vi "15-10-5-2.vi"() -> ()   [LabVIEW 2025]
uses:
  <vilib>/Platform/TimedLoop/XDataNode/timing_clust.ctl
  <vilib>/Platform/TimedLoop/XDataNode/nitl_modes.ctl
  <vilib>/Platform/TimedLoop/XDataNode/wakeup.ctl
  <vilib>/rvi/Emulation/niFpgaSctlEmulationGetInTimedLoop.vi
  <vilib>/rvi/Emulation/niFpgaEmulationReportErrorSimple.vi
  <vilib>/rvi/Emulation/niFpgaGetClockAttributes.vi
  <vilib>/rvi/Emulation/niFpgaCriticalErrorInLSC.vi
  <vilib>/rvi/linearAlgebra/MatrixMultiply/simVIs/SubVI/nifxpla_MatrixMultiply_SimMatrixSizes.vi
  <vilib>/rvi/linearAlgebra/MatrixMultiply/simVIs/SubVI/nifxpla_MatrixMultiply_Sim4WireAdapterVector.vi
  <vilib>/rvi/linearAlgebra/MatrixMultiply/simVIs/SubVI/nifxpla_MatrixMultiply_SimFrameHandShake.vi
  <vilib>/rvi/linearAlgebra/MatrixMultiply/simVIs/SubVI/nifxpla_MatrixMultiply_SimEndlessCounter.vi
  <vilib>/rvi/linearAlgebra/MatrixMultiply/simVIs/SubVI/nifxpla_MatrixMultiply_SimVectorDataBuffer.vi
  <vilib>/rvi/ClientSDK/Core/DevComputerLib/Private/Multiply(dfxp64).vi
  <vilib>/rvi/ClientSDK/Core/DevComputerLib/Private/Dfxp128ToDfxp256.vi
  <vilib>/rvi/ClientSDK/Core/DevComputerLib/Private/Add(dfxp256).vi
  <vilib>/rvi/ClientSDK/Core/DevComputerLib/Private/Subtract(dfxp256).vi
  <vilib>/rvi/ClientSDK/Core/DevComputerLib/Private/ToDfxp64(dfxp256).vi
  <vilib>/platform/TimedLoop/XDataNode/XDataNode.xnode
  <vilib>/rvi/linearAlgebra/MatrixMultiply/XNode/nifxpla_MatrixMultiply.xnode
  <vilib>/rvi/linearAlgebra/MatrixMultiply/simVIs/nifxpla_MatrixMultiply_SimTemplateEinEout.vi
  <vilib>/rvi/linearAlgebra/MatrixMultiply/simVIs/nifxpla_MatrixMultiply_SimTemplateEinVout.vi
  <vilib>/rvi/linearAlgebra/MatrixMultiply/simVIs/nifxpla_MatrixMultiply_SimTemplateVinEout.vi
  <vilib>/rvi/linearAlgebra/MatrixMultiply/simVIs/nifxpla_MatrixMultiply_SimTemplateVinVout.vi
  <vilib>/Platform/TimedLoop/XDataNode/XDNodeRunTimeDep.lvlib
panel:
  out "Latency":u32
  out "Cycle Count 3":i32
  out "C3":fxp<+/-,32,16>[](array[numeric])
  out "C3+B":fxp<+/-,33,17>[](array[numeric])
  out "Cycle Count 2":i32
  out "C2":fxp<+/-,32,16>[](array[numeric])
  out "C2+B":fxp<+/-,33,17>[](array[numeric])
  out "Cycle Count":i32
  out "C1":fxp<+/-,32,16>[](array[numeric])
  out "C1+B":fxp<+/-,33,17>[](array[numeric])
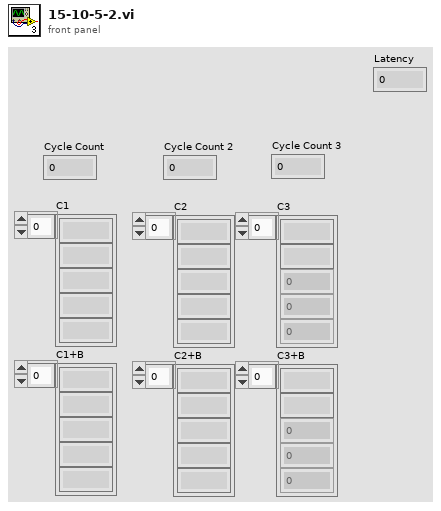
[diagram p1: front panel]
types:
  T1 = typedef "XDNodeRunTimeDep.lvlib/timing_clust.ctl" = cluster{"Expected End [f-1]":u64, "Actual End [f-1]":u64, "Finished Late? [f-1]":bool, "Expected End [i-1]":u64, "Actual End [i-1]":u64, "Finished Late? [i-1]":bool, "Expected Start [i]":u64, "Actual Start [i]":u64, "Expected Start [f]":u64, "Actual Start [f]":u64, "Source Name":string, "Structure Name":string, "Period":i64, "Deadline":i64, "Offset":i64, "Start":i64, "Priority":i32, "Timeout":i32, "Mode":T2, "Wakeup Reason":T3, "Error":errorcluster, "Source Type":string, "Secondary Source Type":string, "Global End Time":u64, "Global Start Time":u64, "Frame Duration":u64, "Iteration Duration":u64, "Assigned CPU":i32, "I/O Scan Engine Mode":u32}
  T2 = typedef "XDNodeRunTimeDep.lvlib/nitl_modes.ctl" = enum32{"No Change", "Process missed periods, maintain original phase", "Discard missed periods, maintain original phase", "Process missed periods, ignore original phase", "Discard missed periods, ignore original phase"}
  T3 = typedef "XDNodeRunTimeDep.lvlib/wakeup.ctl" = enum32{"Normal", "Aborted", "Asynchronous wakeup", "Timing source error", "Timed loop error", "Timeout"}
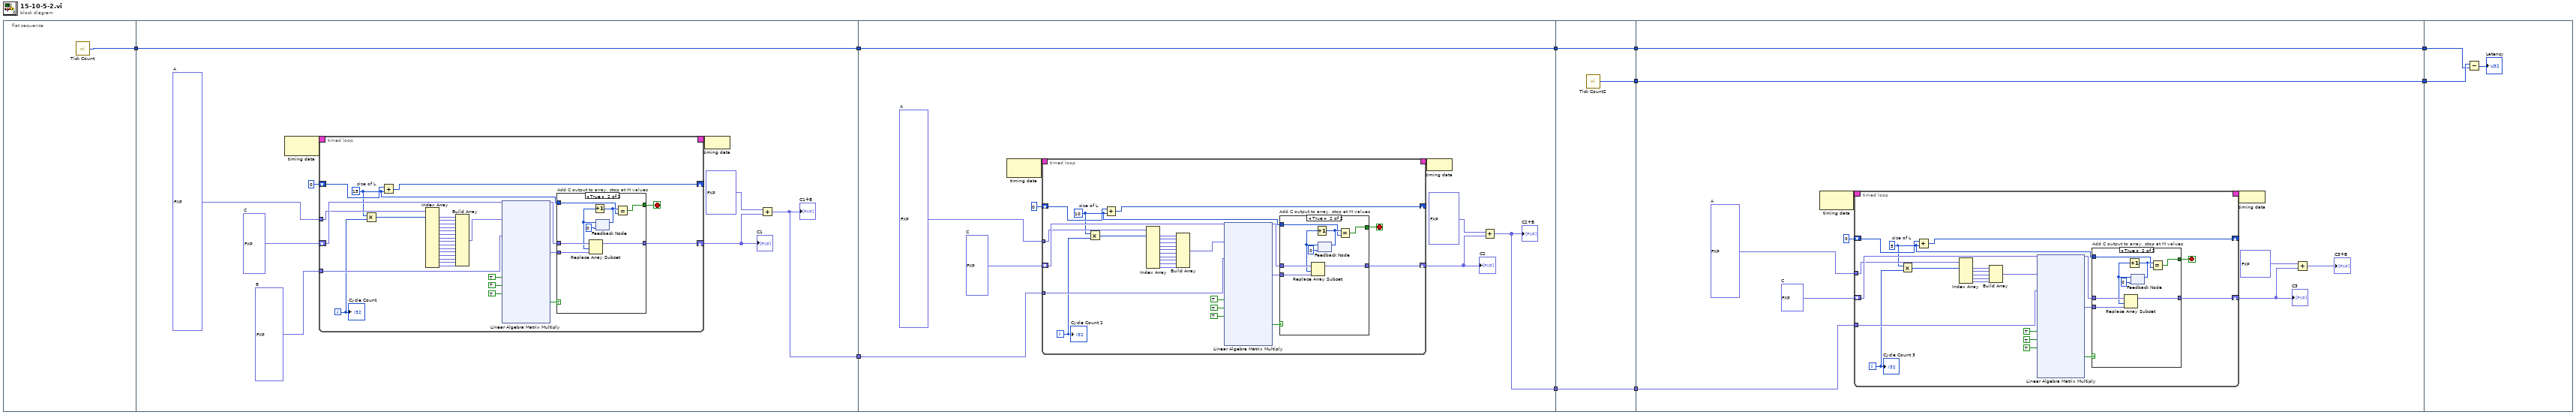
[diagram p0: block diagram]
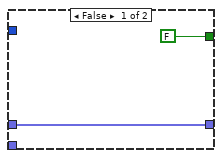
[diagram p2: hidden frame]
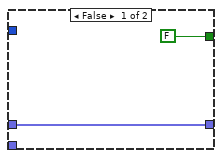
[diagram p3: hidden frame]
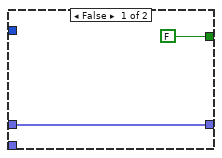
[diagram p4: hidden frame]
diagram:
  n1 = flat-sequence {
    tunnel: [w11] -> w10
    tunnel: [w13] -> w9
    tunnel: [w12] -> w8
    tunnel: w10 -> [w12]
    tunnel: w9 -> [w69]
    tunnel: [w68] -> w7
    tunnel: w8 -> [w67]
    tunnel: [w67] -> w6
    tunnel: w7 -> [w119]
    tunnel: [w119] -> w5
    tunnel: w6 -> [w118]
    tunnel: [w118] -> w4
    tunnel: [w117] -> w3
    tunnel: w5 -> [w122]
    tunnel: w4 -> [w121]
    tunnel: [w121] -> w2
    tunnel: [w120] -> w1
    tunnel: w3 -> [w120]
    tunnel: w2 -> [w167]
    tunnel: w1 -> [w168]
    frame #0 {
      n2 = call "Tick Count"() -> ("Tick Count(Ticks)"=w11:u32)
    }
    frame #1 {
      w17 = fxp<+/-,32,16>[] [0.0, 0.0, 0.0, 0.0, 0.0, 0.0, 0.0, 0.0, 0.0, 0.0, 0.0, 0.0, 0.0, 0.0, 0.0, 0.0, 0.0, 0.0, 0.0, 0.0, 0.0, 0.0, 0.0, 0.0, 0.0, 0.0, 0.0, 0.0, 0.0, 0.0, 0.0, 0.0, 0.0, 0.0, 0.0, 0.0, 0.0, 0.0, 0.0, 0.0, 0.0, 0.0, 0.0, 0.0, 0.0, 0.0, 0.0, 0.0, 0.0, 0.0, 0.0, 0.0, 0.0, 0.0, 0.0, 0.0, 0.0, 0.0, 0.0, 0.0, 0.0, 0.0, 0.0, 0.0, 0.0, 0.0, 0.0, 0.0, 0.0, 0.0, 0.0, 0.0, 0.0, 0.0, 0.0, 0.0, 0.0, 0.0, 0.0, 0.0, 0.0, 0.0, 0.0, 0.0, 0.0, 0.0, 0.0, 0.0, 0.0, 0.0, 0.0, 0.0, 0.0, 0.0, 0.0, 0.0, 0.0, 0.0, 0.0, 0.0, 0.0, 0.0, 0.0, 0.0, 0.0, 0.0, 0.0, 0.0, 0.0, 0.0, 0.0, 0.0, 0.0, 0.0, 0.0, 0.0, 0.0, 0.0, 0.0, 0.0, 0.0, 0.0, 0.0, 0.0, 0.0, 0.0, 0.0, 0.0, 0.0, 0.0, 0.0, 0.0, 0.0, 0.0, 0.0, 0.0, 0.0, 0.0, 0.0, 0.0, 0.0, 0.0, 0.0, 0.0, 0.0, 0.0, 0.0, 0.0, 0.0, 0.0]  # A
      w18 = fxp<+/-,32,16>[] [0.0, 0.0, 0.0, 0.0, 0.0, 0.0, 0.0, 0.0, 0.0, 0.0, 0.0, 0.0, 0.0, 0.0, 0.0]  # B
      w19 = fxp<+/-,32,16>[] [0.0, 0.0, 0.0, 0.0, 0.0, 0.0, 0.0, 0.0, 0.0, 0.0]  # C
      n3 = node-c288() -> (w21:T1)  [unwired: 1 in]
      n4 = timed-loop {
        timing: w21 -> [_]
        timing-out: [_] -> w20
        shift-right: [w51] -> w15
        shift-left: w19 -> [w50]
        tunnel: w18 -> [w47]
        tunnel: w17 -> [w30]
        shift-right: [w43] -> _
        shift-left: 0 ("length") -> [w44]
        i -> [w29]
        stop <- w49 stop-if-true
        w28 = 15  # size of L
        n5 = Multiply(x=w28, y=w29) -> (x*y=w41:i32)
        n6 = Add(x=w44, y=w28) -> (x+y=w43:i32)
        n7 = Index Array(array=w30, index #1=w41) -> (element #1=w40:fxp<+/-,32,16>, element #2=w39:fxp<+/-,32,16>, element #3=w38:fxp<+/-,32,16>, element #4=w37:fxp<+/-,32,16>, element #5=w36:fxp<+/-,32,16>, element #6=w35:fxp<+/-,32,16>, element #7=w34:fxp<+/-,32,16>, element #8=w33:fxp<+/-,32,16>, element #9=w32:fxp<+/-,32,16>, element #10=w31:fxp<+/-,32,16>, element #11=w26:fxp<+/-,32,16>, element #12=w25:fxp<+/-,32,16>, element #13=w24:fxp<+/-,32,16>, element #14=w23:fxp<+/-,32,16>, element #15=w22:fxp<+/-,32,16>)  [unwired: 14 in]
        n8 = Build Array(w40, w39, w38, w37, w36, w35, w34, w33, w32, w31, w26, w25, w24, w23, w22) -> (w27:fxp<+/-,32,16>[])
        n9 = xnode ("Linear Algebra Matrix Multiply")("ar"=w27, "br"=w47, "a valid"=TRUE, "b valid"=TRUE, "ready for output (T)"=TRUE) -> ("cr"=w46:fxp<+/-,64,36>[], "output valid"=w42:bool)  [unwired: 2 in, 4 out]
        n10 = case "Add C output to array, stop at M values" shown="True" w42 {
          tunnel: w46 -> [_ w58]
          tunnel: [w54 w61] -> w51
          tunnel: w50 -> [w54 w62]
          tunnel: [FALSE w59] -> w49
          tunnel: w28 -> [_ w55]
          frame False {
          }
          frame True {
            n11 = feedback #1(0 ("x")) -> (w57:i32)
            n12 = Replace Array Subset(array=w62, new element=w58, index=w57) -> (w61:fxp<+/-,32,16>[])
            n13 = Increment(x=w57) -> (x+1=w56:i32)
            n14 = feedback-in #1(w56) -> ()
            n15 = Equal?(x=w56, y=w55) -> (x = y?=w59:bool)
          }
        }
        "Cycle Count" <- w29
      }
      "C1" <- w15
      n16 = node-c288(w20) -> ()
      n17 = Add(x=fxp<+/-,32,16>[] [0.5, 0.5, 0.5, 0.5, 0.5, 0.0, 0.0, 0.0, 0.0, 0.0], y=w15) -> (x+y=w13:fxp<+/-,33,17>[])
      "C1+B" <- w13
    }
    frame #2 {
      w73 = fxp<+/-,32,16>[] [0.0, 0.0, 0.0, 0.0, 0.0, 0.0, 0.0, 0.0, 0.0, 0.0, 0.0, 0.0, 0.0, 0.0, 0.0, 0.0, 0.0, 0.0, 0.0, 0.0, 0.0, 0.0, 0.0, 0.0, 0.0, 0.0, 0.0, 0.0, 0.0, 0.0, 0.0, 0.0, 0.0, 0.0, 0.0, 0.0, 0.0, 0.0, 0.0, 0.0, 0.0, 0.0, 0.0, 0.0, 0.0, 0.0, 0.0, 0.0, 0.0, 0.0]  # A
      w74 = fxp<+/-,32,16>[] [0.0, 0.0, 0.0, 0.0, 0.0]  # C
      n18 = node-c288() -> (w76:T1)  [unwired: 1 in]
      n19 = timed-loop {
        timing: w76 -> [_]
        timing-out: [_] -> w75
        shift-right: [w101] -> w71
        shift-left: w74 -> [w100]
        tunnel: w69 -> [w97]
        tunnel: w73 -> [w85]
        shift-right: [w93] -> _
        shift-left: 0 ("length") -> [w94]
        i -> [w84]
        stop <- w99 stop-if-true
        w83 = 10  # size of L
        n20 = Multiply(x=w83, y=w84) -> (x*y=w91:i32)
        n21 = Add(x=w94, y=w83) -> (x+y=w93:i32)
        n22 = Index Array(array=w85, index #1=w91) -> (element #1=w90:fxp<+/-,32,16>, element #2=w89:fxp<+/-,32,16>, element #3=w88:fxp<+/-,32,16>, element #4=w87:fxp<+/-,32,16>, element #5=w86:fxp<+/-,32,16>, element #6=w81:fxp<+/-,32,16>, element #7=w80:fxp<+/-,32,16>, element #8=w79:fxp<+/-,32,16>, element #9=w78:fxp<+/-,32,16>, element #10=w77:fxp<+/-,32,16>)  [unwired: 9 in]
        n23 = Build Array(w90, w89, w88, w87, w86, w81, w80, w79, w78, w77) -> (w82:fxp<+/-,32,16>[])
        n24 = xnode ("Linear Algebra Matrix Multiply")("ar"=w82, "br"=w97, "a valid"=TRUE, "b valid"=TRUE, "ready for output (T)"=TRUE) -> ("cr"=w96:fxp<+/-,64,37>[], "output valid"=w92:bool)  [unwired: 2 in, 4 out]
        n25 = case "Add C output to array, stop at M values" shown="True" w92 {
          tunnel: w96 -> [_ w108]
          tunnel: [w104 w111] -> w101
          tunnel: w100 -> [w104 w112]
          tunnel: [FALSE w109] -> w99
          tunnel: w83 -> [_ w105]
          frame False {
          }
          frame True {
            n26 = feedback #2(0 ("x")) -> (w107:i32)
            n27 = Replace Array Subset(array=w112, new element=w108, index=w107) -> (w111:fxp<+/-,32,16>[])
            n28 = Increment(x=w107) -> (x+1=w106:i32)
            n29 = feedback-in #2(w106) -> ()
            n30 = Equal?(x=w106, y=w105) -> (x = y?=w109:bool)
          }
        }
        "Cycle Count 2" <- w84
      }
      "C2" <- w71
      n31 = node-c288(w75) -> ()
      n32 = Add(x=fxp<+/-,32,16>[] [0.5, 0.5, 0.5, 0.5, 0.5], y=w71) -> (x+y=w68:fxp<+/-,33,17>[])
      "C2+B" <- w68
    }
    frame #3 {
      n33 = call "Tick Count2"() -> ("Tick Count(Ticks)"=w117:u32)
    }
    frame #4 {
      w127 = fxp<+/-,32,16>[] [0.0, 0.0, 0.0, 0.0, 0.0, 0.0, 0.0, 0.0, 0.0, 0.0]  # A
      w128 = fxp<+/-,32,16>[] [0.0, 0.0]  # C
      n34 = node-c288() -> (w130:T1)  [unwired: 1 in]
      n35 = timed-loop {
        timing: w130 -> [_]
        timing-out: [_] -> w129
        shift-right: [w150] -> w125
        shift-left: w128 -> [w149]
        tunnel: w122 -> [w146]
        tunnel: w127 -> [w134]
        shift-right: [w142] -> _
        shift-left: 0 ("length") -> [w143]
        i -> [w133]
        stop <- w148 stop-if-true
        w132 = 5  # size of L
        n36 = Multiply(x=w132, y=w133) -> (x*y=w140:i32)
        n37 = Add(x=w143, y=w132) -> (x+y=w142:i32)
        n38 = Index Array(array=w134, index #1=w140) -> (element #1=w139:fxp<+/-,32,16>, element #2=w138:fxp<+/-,32,16>, element #3=w137:fxp<+/-,32,16>, element #4=w136:fxp<+/-,32,16>, element #5=w135:fxp<+/-,32,16>)  [unwired: 4 in]
        n39 = Build Array(w139, w138, w137, w136, w135) -> (w131:fxp<+/-,32,16>[])
        n40 = xnode ("Linear Algebra Matrix Multiply")("ar"=w131, "br"=w146, "a valid"=TRUE, "b valid"=TRUE, "ready for output (T)"=TRUE) -> ("cr"=w145:fxp<+/-,64,36>[], "output valid"=w141:bool)  [unwired: 2 in, 4 out]
        n41 = case "Add C output to array, stop at M values" shown="True" w141 {
          tunnel: w145 -> [_ w157]
          tunnel: [w153 w160] -> w150
          tunnel: w149 -> [w153 w161]
          tunnel: [FALSE w158] -> w148
          tunnel: w132 -> [_ w154]
          frame False {
          }
          frame True {
            n42 = feedback #3(0 ("x")) -> (w156:i32)
            n43 = Replace Array Subset(array=w161, new element=w157, index=w156) -> (w160:fxp<+/-,32,16>[])
            n44 = Increment(x=w156) -> (x+1=w155:i32)
            n45 = feedback-in #3(w155) -> ()
            n46 = Equal?(x=w155, y=w154) -> (x = y?=w158:bool)
          }
        }
        "Cycle Count 3" <- w133
      }
      "C3" <- w125
      n47 = node-c288(w129) -> ()
      n48 = Add(x=fxp<+/-,32,16>[] [0.5, 0.5], y=w125) -> (x+y=→"C3+B":fxp<+/-,33,17>[])
    }
    frame #5 {
      n49 = Subtract(x=w168, y=w167) -> (x-y=→"Latency":u32)
    }
  }
